vi "Networkstream UI Command.vi"(8 "error in":errorcluster, 10 "Data":variant, 11 "Message":string) -> (0 "error out":errorcluster)   [LabVIEW 2022 SP3]
uses:
  Global 1.vi
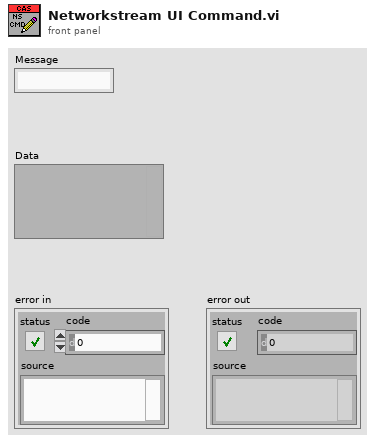
[diagram p1: front panel]
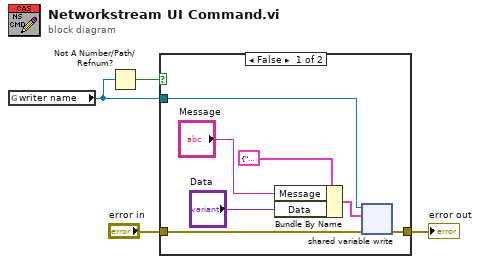
[diagram p0: block diagram]
diagram:
  n1 = global read "Global 1.vi" "writer name"() -> (w1:refnum<k21>)
  n2 = Not A Number/Path/Refnum?(number/path/refnum=w1) -> (NaN/Path/Refnum?=w4:bool)
  n3 = case shown="False" w4 {
    tunnel: w1 -> [w11 _]
    tunnel: "error in" -> [w6 w12]
    tunnel: [w5 w12] -> w2
    frame False {
      n4 = Bundle By Name(cluster=cluster{"Message":string, "Data":variant} {"Message"="", "Data"=variant}, "Message"="Message", "Data"="Data") -> (w10:cluster{"Message":string, "Data":variant})
      n5 = shared-variable-write(w11, w6, w10) -> (w5:errorcluster)  [unwired: 1 in, 2 out]
    }
    frame True {
    }
  }
  "error out" <- w2
